vi "概率密度.vi"() -> ()   [LabVIEW 2018]
uses:
  <vilib>/gmath/statdist.llb/Cauchy PDF.vi
  <vilib>/gmath/NI_Gmath.lvlib
panel:
  in  "a":dbl
  in  "停止":bool
  out "pdf(x)":dbl=0.3183098861837907
  in  "b":dbl=1.0
  in  "x":dbl
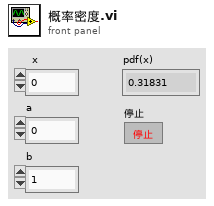
[diagram p1: front panel]
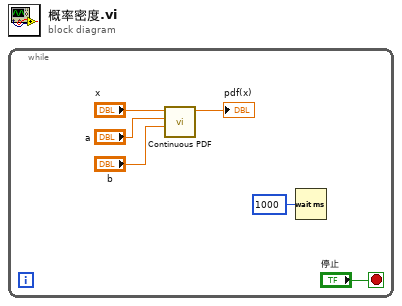
[diagram p0: block diagram]
diagram:
  n1 = while {
    stop <- "停止" stop-if-true
    n2 = call-poly <vilib>:"Continuous PDF.vi"("b"="b", "a"="a", "x"="x") -> ("pdf(x)"=→"pdf(x)":dbl)  [unwired: 7 in, 1 out]
    n3 = Wait (ms)(milliseconds to wait=u32 1000 ("等待时间（毫秒）")) -> ()  [unwired: 1 out]
  }
